vi "tp3-3.vi"() -> ()   [LabVIEW 2013]
uses:
  <vilib>/sound2/lvsound2.llb/Sound Input Read (DBL).vi
panel:
  out "Boolean":bool
  in  "stop":bool
  out "Waveform Graph":dbl[](graph)
  in  "Cluster":T1={"Sample rate S/s"=44100.0, "Number of channels"=1.0, "bits per sample"=16.0}
  in  "Buffer de lectura":dbl=11025.0
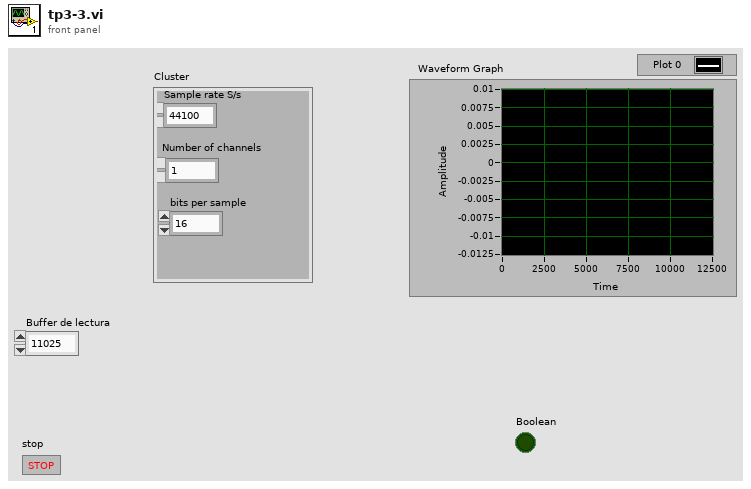
[diagram p1: front panel]
types:
  T1 = cluster{"Sample rate S/s":dbl, "Number of channels":dbl, "bits per sample":dbl}
  T2 = typedef "Sound Input Task ID.ctl" = u32
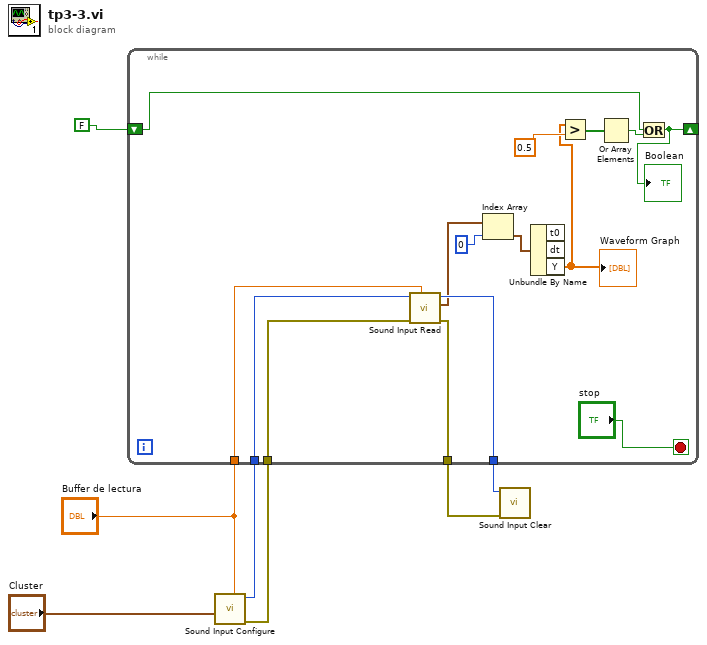
[diagram p0: block diagram]
diagram:
  n1 = call <vilib>:"Sound Input Configure.vi"("number of samples/ch"="Buffer de lectura", "sound format"="Cluster") -> ("error out"=w6:errorcluster, "task ID"=w5:T2)  [unwired: 8 in]
  n2 = while {
    tunnel: [w22] -> w7
    tunnel: w6 -> [w21]
    tunnel: w5 -> [w20]
    tunnel: [w19] -> w4
    tunnel: "Buffer de lectura" -> [w18]
    shift-right: [w8] -> _
    shift-left: FALSE -> [w9]
    stop <- "stop" stop-if-true
    n3 = call-poly <vilib>:"Sound Input Read.vi"("number of samples/ch"=w18, "error in (no error)"=w21, "task ID"=w20) -> ("error out"=w22:errorcluster, "data"=w17:waveform(dbl)[], "task ID out"=w19:T2)  [unwired: 6 in]
    n4 = Index Array(array=w17, index=0) -> (element=w15:waveform(dbl))
    n5 = Unbundle By Name(w15) -> ("Y"=w11:dbl[])  [unwired: 2 out]
    "Waveform Graph" <- w11
    n6 = Greater?(x=w11, y=0.5) -> (0:w12:bool[])
    n7 = Or Array Elements(Boolean array=w12) -> (logical OR=w10:bool)
    n8 = Or(x=w9, y=w10) -> (x .or. y?=w8:bool)
    "Boolean" <- w8
  }
  n9 = call <vilib>:"Sound Input Clear.vi"("error in (no error)"=w7, "task ID"=w4) -> ()  [unwired: 9 in, 1 out]
